vi "execute.vi"(8 "error in (no error)":errorcluster, 11 "SellStock in":refnum<class "SellStock.lvclass">) -> (0 "error out":errorcluster, 3 "SellStock out":refnum<class "SellStock.lvclass">)   [LabVIEW 2016, in "SellStock.lvclass"]
uses:
  SellStock.lvclass
  SellStock.lvclass/SellStock.ctl
  Stock Class/Stock.lvclass
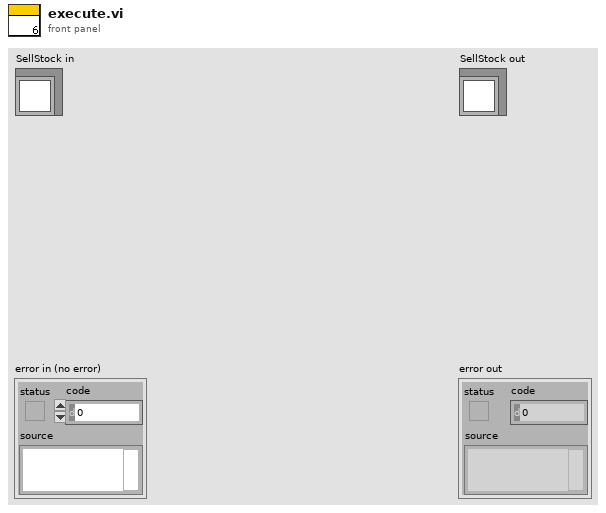
[diagram p1: front panel]
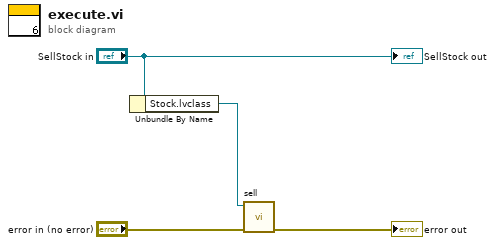
[diagram p0: block diagram]
diagram:
  n1 = Unbundle By Name("SellStock in") -> ("Stock.lvclass"=w1:refnum<class "Stock.lvclass">)
  n2 = call "sell.vi"("error in (no error)"="error in (no error)", "Stock in"=w1) -> ("error out"=→"error out":errorcluster)  [unwired: 8 in, 1 out]
  "SellStock out" <- "SellStock in"
